vi "Counter.vi"(6 "Reset Counter":bool, 7 "Counter Parameters":T1={"Edge"=enum."Rising Edge", "Gate?"=FALSE, "Count Direction"=enum."Count Up", "Terminal Count"=16777216, "Ticks to Filter"=2, "High Pulse Time (us)"=1000}, 8 "Run?":bool=TRUE, 10 "Ctr Gate":bool, 11 "Ctr Source":bool) -> (2 "Ctr Out":bool, 3 "Counter Register":u64)   [LabVIEW 2010]
uses:
  <userlib>/_NI VeriStand FPGA Support/NI VeriStand RIO Library/IP Based IO/Counter/common/CounterControl.ctl
panel:
  # "ON"
  # "OFF"
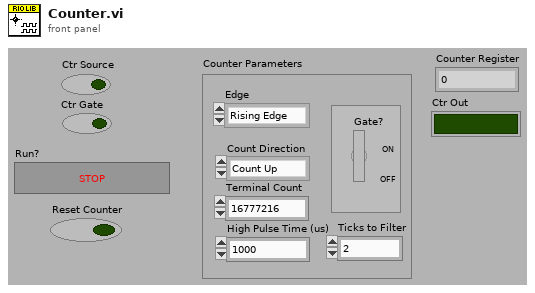
[diagram p1: front panel]
types:
  T1 = typedef "CounterControl.ctl" = cluster{"Edge":enum16{"Falling Edge", "Rising Edge"}, "Gate?":bool, "Count Direction":enum16{"Count Up", "Count Down"}, "Terminal Count":u64, "Ticks to Filter":u32, "High Pulse Time (us)":u32}
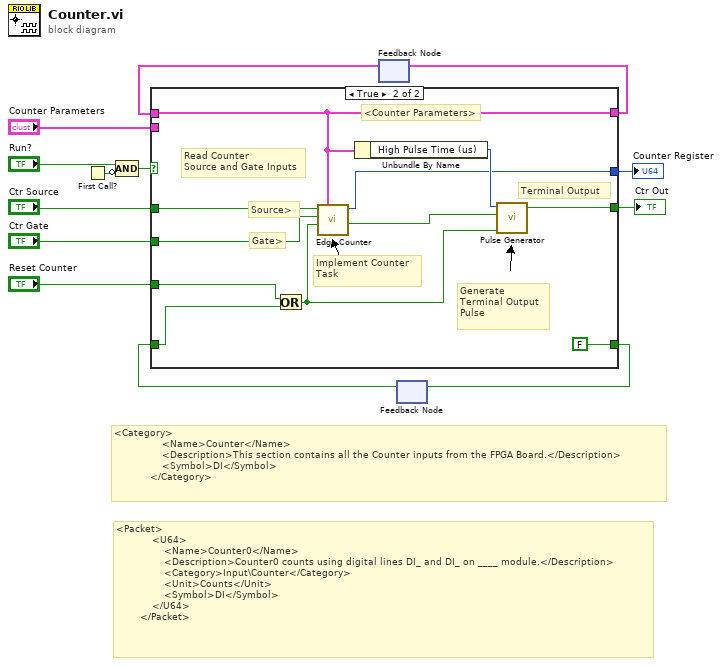
[diagram p0: block diagram]
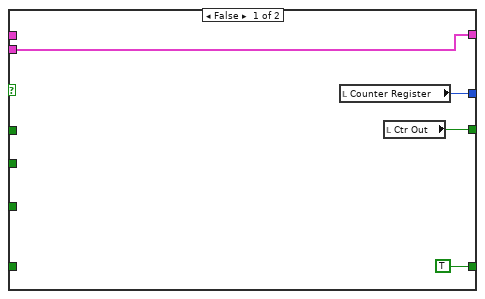
[diagram p2: hidden frame]
diagram:
  # "<Category>\n                <Name>Counter</Name>\n                <Description>This section contains all the Counter inputs from the FPGA Board.</Description>\n                <Symbol>DI</Symbol>\n            </Category>"
  # "<Packet>\n            <U64>\n                <Name>Counter0</Name>\n                <Description>Counter0 counts using digital lines DI_ and DI_ on ____ module.</Description>\n                <Category>Input\\Counter</Category>\n                <Unit>Counts</Unit>\n                <Symbol>DI</Symbol>\n            </U64>\n        </Packet>"
  n1 = First Call?() -> (First Call?: T/F=w3:bool)
  n2 = Compound Arithmetic op=AND("Run?", invert w3) -> (w1:bool)
  n3 = feedback #1() -> (w10:T1)  [unwired: 1 in]
  n4 = feedback #2() -> (w12:bool)  [unwired: 1 in]
  n5 = case shown="True" w1 {
    tunnel: w10 -> [_ w27]
    tunnel: [w15 w27] -> w11
    tunnel: w12 -> [_ w25]
    tunnel: [TRUE FALSE] -> w13
    tunnel: "Ctr Source" -> [_ w22]
    tunnel: "Ctr Gate" -> [_ w21]
    tunnel: "Reset Counter" -> [_ w20]
    tunnel: [w16 w19] -> w6
    tunnel: "Counter Parameters" -> [w15 _]
    tunnel: [w14 w18] -> w4
    frame False {
      n6 = local read "Counter Register"() -> (w14:u64)
      n7 = local read "Ctr Out"() -> (w16:bool)
    }
    frame True {
      # "Read Counter\nSource and Gate Inputs"
      # "<Counter Parameters>"
      # "Generate\nTerminal Output\nPulse"
      # "Implement Counter\nTask"
      # "Terminal Output"
      # "Gate>"
      # "Source>"
      n8 = Or(x=w20, y=w25) -> (x .or. y?=w23:bool)
      n9 = call <userlib>:"Edge Counter.vi"("Counter Parameters"=w27, "Reset Counter"=w23, "Gate Input"=w21, "Ctr Source"=w22) -> ("Terminal Count?"=w26:bool, "Counter Register"=w18:u64)  [unwired: 6 in]
      n10 = Unbundle By Name(w27) -> ("High Pulse Time (us)"=w28:u32)
      n11 = call <userlib>:"Pulse Generator.vi"("Reset Counter"=w23, "Terminal Count?"=w26, "High Pulse Time"=w28) -> ("CtrOut"=w19:bool)  [unwired: 2 in, 1 out]
    }
  }
  "Ctr Out" <- w6
  "Counter Register" <- w4
  n12 = feedback-in #1(w11) -> ()
  n13 = feedback-in #2(w13) -> ()
